vi "Color Ramp Change Display Format.vi"(8 "Error In":errorcluster, 11 "ColorRamp Refnum":refnum<vi>) -> (0 "Error Out":errorcluster)   [LabVIEW 2021, in "Palette.lvlib"]
uses:
  Palette.lvlib
  GUI/GUI.lvlib
panel:
  # "see the License on the block diagram (Ctrl+E or Window:Show Block Diagram)"
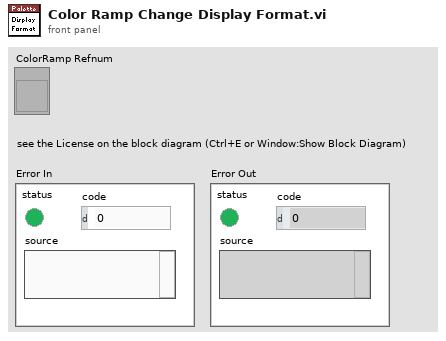
[diagram p1: front panel]
types:
  T1 = typedef "LVFormatAndPrecisionTypeDef.ctl" = cluster{"Format":u8, "Precision":u8}
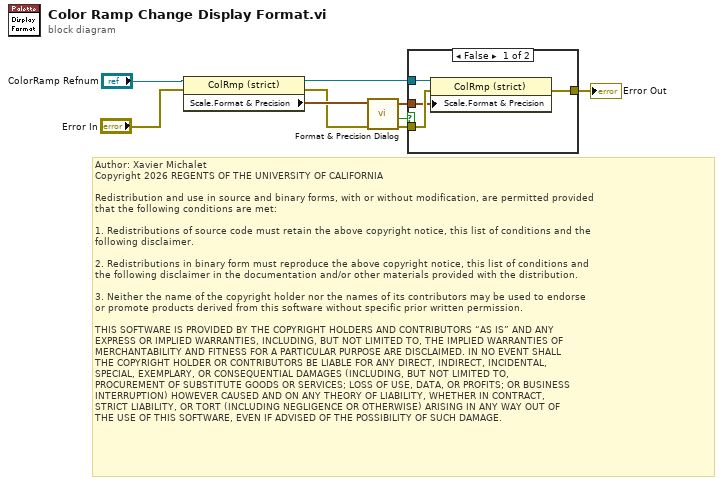
[diagram p0: block diagram]
diagram:
  # "Author: Xavier Michalet\nCopyright 2026 REGENTS OF THE UNIVERSITY OF CALIFORNIA\n\nRedistribution and use in source and binary forms, with or without modification, are permitted provided\nthat the following conditions are met:\n\n1. Redistributions of source code must retain the above copyright notice, this list of conditions and the\nfollowing disclaimer.\n\n2. Redistributions in binary form must reproduce the above copyright notice, this list of conditions and\nthe following disclaimer in the documentation and/or other materials provided with the distribution.\n\n3. Neither the name of the copyright holder nor the names of its contributors may be used to endorse \nor promote products derived from this software without specific prior written permission.\n\nTHIS SOFTWARE IS PROVIDED BY THE COPYRIGHT HOLDERS AND CONTRIBUTORS “AS IS” AND ANY \nEXPRESS OR IMPLIED WARRANTIES, INCLUDING, BUT NOT LIMITED TO, THE IMPLIED WARRANTIES OF\nMERCHANTABILITY AND FITNESS FOR A PARTICULAR PURPOSE ARE DISCLAIMED. IN NO EVENT SHALL\nTHE COPYRIGHT HOLDER OR CONTRIBUTORS BE LIABLE FOR ANY DIRECT, INDIRECT, INCIDENTAL, \nSPECIAL, EXEMPLARY, OR CONSEQUENTIAL DAMAGES (INCLUDING, BUT NOT LIMITED TO, \nPROCUREMENT OF SUBSTITUTE GOODS OR SERVICES; LOSS OF USE, DATA, OR PROFITS; OR BUSINESS\nINTERRUPTION) HOWEVER CAUSED AND ON ANY THEORY OF LIABILITY, WHETHER IN CONTRACT, \nSTRICT LIABILITY, OR TORT (INCLUDING NEGLIGENCE OR OTHERWISE) ARISING IN ANY WAY OUT OF\nTHE USE OF THIS SOFTWARE, EVEN IF ADVISED OF THE POSSIBILITY OF SUCH DAMAGE."
  n1 = property class="ColRmp (strict)"(reference="ColorRamp Refnum", error in="Error In") -> (reference out=w5:refnum<vi>, error out=w2:errorcluster, "Scale.Format & Precision"=w3:T1)
  n2 = call "Format & Precision Dialog.vi"("Error In"=w2, "Display Format in"=w3) -> ("Error Out"=w8:errorcluster, "Cancelled?"=w1:bool, "Display Format out"=w7:T1)  [unwired: 7 in]
  n3 = case shown="False" w1 {
    tunnel: [w13 w14] -> w9
    tunnel: w8 -> [w12 w14]
    tunnel: w7 -> [w11 _]
    tunnel: w5 -> [w10 _]
    frame False {
      n4 = property class="ColRmp (strict)"(reference=w10, error in=w12, "Scale.Format & Precision"=w11) -> (error out=w13:errorcluster)  [unwired: 1 out]
    }
    frame True {
    }
  }
  "Error Out" <- w9
